vi "RT Main.vi"() -> ()   [LabVIEW 2021]
doc: "Demonstrates how to use a dispatcher and message queues to receive data from the host computer."
uses:
  <vilib>/myRIO/Express VI/Onboard Devices/LED/LED Express VI.xnode
  <vilib>/myRIO/Instrument Drivers/Onboard IO/DIO/vis/Write.vi
  <vilib>/myRIO/Instrument Drivers/Onboard IO/DIO/DIO.lvlib
  <vilib>/myRIO/Common/Instrument Driver Framework/myRIO v1.0/DIO/typedefs/DIO Channels Enum.ctl
  <vilib>/myRIO/Common/Instrument Driver Framework/myRIO v1.0/DIO/typedefs/DIO Channels List.ctl
  <vilib>/myRIO/Common/Instrument Driver Framework/Utilities/typedefs/Generic FPGA Reference.ctl
  <vilib>/myRIO/Common/Instrument Driver Framework/Utilities/typedefs/myRIO v1.0 Reference.ctl
  <vilib>/myRIO/Common/Instrument Driver Framework/Utilities/typedefs/Hardware Version Enum.ctl
  <vilib>/myRIO/Common/Instrument Driver Framework/Utilities/typedefs/myRIO Generic Hardware Reference.ctl
  <vilib>/myRIO/Instrument Drivers/Onboard IO/DIO/typedefs/DIO Reference.ctl
  <vilib>/myRIO/Instrument Drivers/Onboard IO/DIO/vis/myRIO DIO Open.xnode
  <vilib>/myRIO/Common/Instrument Driver Framework/Utilities/vis/Is FPGA Ref Available.vi
  <vilib>/myRIO/Common/Instrument Driver Framework/myRIO v1.0/DIO/vis/myRIO v1.1 Open DIO.vi
  <vilib>/userdefined/High Color/nirio_resource_hc.ctl
  <vilib>/myRIO/Instrument Drivers/Utilities/Utilities.lvlib
panel:
  out "LED Status":bool[](array[boolean])
  out "error out":errorcluster
  in  "Stop":bool
  in  "Queue Name":string="Target"
  in  "Local Port":u16=58432
  # "Overview: Demonstrates how to use a dispatcher and message queues to receive data from the host computer. \nInstructions:\n1. Verify if Desktop Main.vi is already running.\n2. Run this VI.\n3. Observe the LEDs on the myRIO device and the value of LED Status on this VI. They change when the value of Tank on Desktop Main.vi changes.\n4. Click Stop to stop this VI."
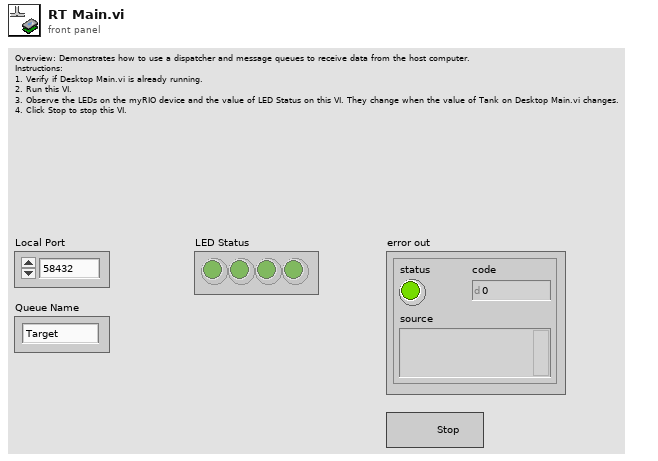
[diagram p1: front panel]
types:
  T1 = typedef "DIO.lvlib/DIO Reference.ctl" = cluster{"myRIO Reference":T2, "DIO Channels List":T6}
  T2 = typedef "myRIO Generic Hardware Reference.ctl" = cluster{"myRIO Model":T3, "myRIO Hardware Reference":T4}
  T3 = typedef "Hardware Version Enum.ctl" = enum16{"Unknown", "myRIO-1900", "myRIO-1950", "roboRIO", "NI ELVIS RIO CM", "ELVIS III"}
  T4 = typedef "myRIO v1.0 Reference.ctl" = cluster{"Generic FPGA Reference":T5, "Allow multiple opens":bool}
  T5 = typedef "Generic FPGA Reference.ctl" = refnum<k20>
  T6 = typedef "DIO Channels List.ctl" = T7[]
  T7 = typedef "DIO Channels Enum.ctl" = enum16{"Not Connected", "C/DIO0", "C/DIO1", "C/DIO2", "C/DIO3", "C/DIO4", "C/DIO5", "C/DIO6", "C/DIO7", "A/DIO0", "A/DIO1", "A/DIO2", "A/DIO3", "A/DIO4", "A/DIO5", "A/DIO6", "A/DIO7", "A/DIO8", "A/DIO9", "A/DIO10", "A/DIO11", "A/DIO12", "A/DIO13", "A/DIO14", "A/DIO15", "A/DIO16", "A/DIO17", "A/DIO18", "A/DIO19", "B/DIO0", "B/DIO1", "B/DIO2", "B/DIO3", "B/DIO4", "B/DIO5", "B/DIO6", "B/DIO7", "B/DIO8", "B/DIO9", "B/DIO10", "B/DIO11", "B/DIO12", "B/DIO13", "B/DIO14", "B/DIO15", "B/DIO16", "B/DIO17", "B/DIO18", "B/DIO19", "LED0", "LED1", "LED2", "LED3", "Button0", "DIO/DIO0", "DIO/DIO1", "DIO/DIO2", "DIO/DIO3", "DIO/DIO4", "DIO/DIO5", "DIO/DIO6", "DIO/DIO7", "DIO/DIO8", "DIO/DIO9", "SPI/CS0", "SPI/CS1", "SPI/CS2", "SPI/CS3", "LED RADIO (Green)", "LED RADIO (Red)", "LED COMM (Green)", "LED COMM (Red)", "LED MODE (Green)", "LED MODE (Red)"}
  T8 = typedef "nirio_resource_hc.ctl" = tag
  T9 = typedef "Message.ctl" = cluster{"Name":string, "Value":string, "Local IP":string, "Local Queue":string, "Remote IP":string, "Remote Queue":string}
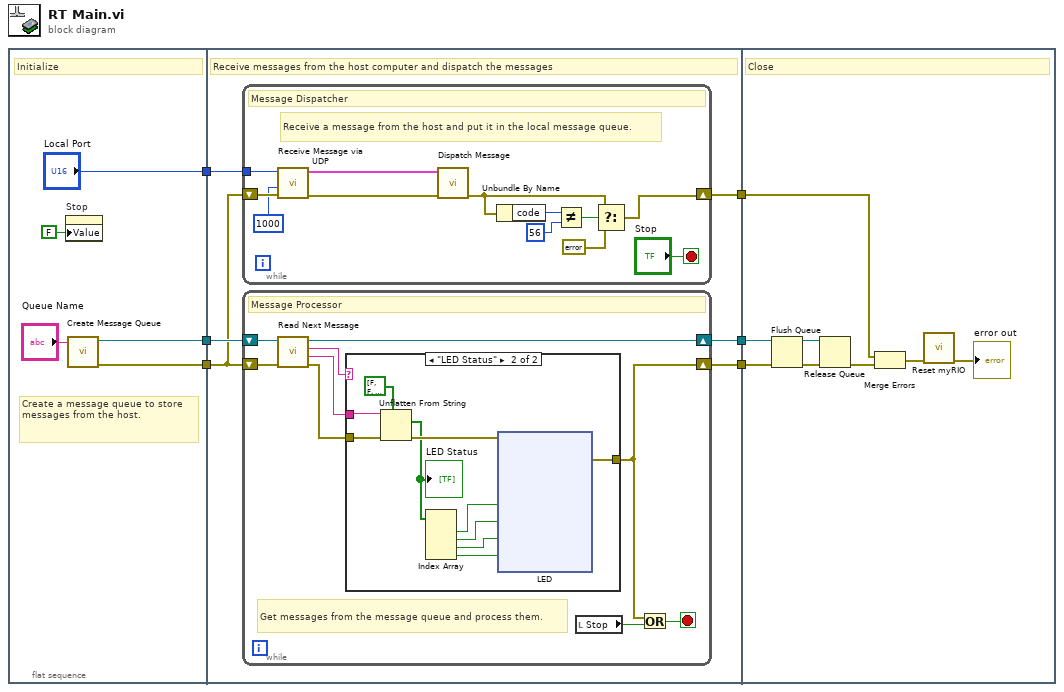
[diagram p0: block diagram]
diagram:
  n1 = flat-sequence {
    tunnel: [w10] -> w6
    tunnel: ["Local Port"] -> w3
    tunnel: [w8] -> w1
    tunnel: w6 -> [w15]
    tunnel: [w17] -> w5
    tunnel: [w16] -> w4
    tunnel: w3 -> [w14]
    tunnel: [w13] -> w2
    tunnel: w1 -> [w12]
    tunnel: w5 -> [w95]
    tunnel: w4 -> [w92]
    tunnel: w2 -> [w90]
    frame #0 {
      # "Create a message queue to store messages from the host."
      # "Initialize"
      n2 = property on="Stop" class="Bool (strict)"("Value"=FALSE ("Stop Button")) -> ()  [unwired: 2 in, 2 out]
      n3 = call "Create Message Queue.vi"("queue name"="Queue Name") -> ("error out"=w8:errorcluster, "Message queue"=w10:refnum<queue>)  [unwired: 9 in]
    }
    frame #1 {
      # "Receive messages from the host computer and dispatch the messages"
      n4 = while {
        shift-right: [w77] -> w13
        shift-left: w12 -> [w86]
        tunnel: w14 -> [w85]
        stop <- "Stop" stop-if-true
        # "Receive a message from the host and put it in the local message queue."
        # "Message Dispatcher"
        n5 = call "Receive Message via UDP.vi"("error in"=w86, "timeout ms (25000)"=1000, "Local Port"=w85) -> ("error out"=w83:errorcluster, "Message"=w84:T9)  [unwired: 7 in]
        n6 = call "Dispatch Message.vi"("error in"=w83, "Message"=w84) -> ("error out"=w78:errorcluster)  [unwired: 8 in, 1 out]
        n7 = Unbundle By Name(w78) -> ("code"=w81:i32)
        n8 = Not Equal?(x=w81, y=56) -> (x != y?=w82:bool)
        n9 = Select(t=w78, s=w82, f=errorcluster {"status"=FALSE, "code"=0, "source"=""} ("error out")) -> (s? t:f=w77:errorcluster)
      }
      n10 = while {
        shift-right: [w20] -> w16
        shift-left: w12 -> [w25]
        shift-right: [w24] -> w17
        shift-left: w15 -> [w26]
        stop <- w19 stop-if-true
        # "Get messages from the message queue and process them."
        # "Message Processor"
        n11 = call "Read Next Message.vi"("error in"=w25, "Message queue"=w26) -> ("error out"=w23:errorcluster, "Message Value"=w21:string, "Message Name"=w22:string, "Message queue out"=w24:refnum<queue>)  [unwired: 6 in]
        n12 = case shown="\"LED Status\"" w22 {
          tunnel: w23 -> [w27 w30]
          tunnel: [w27 w28] -> w20
          tunnel: w21 -> [_ w32]
          frame Default {
          }
          frame "LED Status" {
            n13 = Unflatten From String(type=bool[] [FALSE, FALSE, FALSE, FALSE] ("LED Status"), binary string=w32, error in (no error)=w30) -> (value=w29:bool[], error out=w37:errorcluster)  [unwired: 2 in, 1 out]
            "LED Status" <- w29
            n14 = Index Array(array=w29) -> (element #1=w36:bool, element #2=w35:bool, element #3=w34:bool, element #4=w33:bool)  [unwired: 4 in]
            n15 = xnode "LED"("LED0"=w36, "LED1"=w35, "LED2"=w34, "LED3"=w33, "error in (no error)"=w37) -> ("error out"=w28:errorcluster)
          }
        }
        n16 = local read "Stop"() -> (w18:bool)
        n17 = Or(x=w20, y=w18) -> (x .or. y?=w19:bool)
      }
    }
    frame #2 {
      # "Close"
      n18 = Flush Queue(queue=w95, error in (no error)=w92) -> (queue out=w93:refnum<queue>, error out=w94:errorcluster)  [unwired: 1 out]
      n19 = Release Queue(queue=w93, error in (no error)=w94) -> (error out=w91:errorcluster)  [unwired: 1 in, 2 out]
      n20 = Merge Errors(w90, w91) -> (w89:errorcluster)
      n21 = call <vilib>:"Reset myRIO.vi"("error in (no error)"=w89) -> ("error out"=→"error out":errorcluster)  [unwired: 10 in]
    }
  }
